vi "ISS Main.vi"() -> ()   [LabVIEW 2014]
uses:
  <vilib>/Instr/_visa.llb/VISA Configure Serial Port (Instr).vi
  controls/scan data action.ctl
  controls/main states.ctl
  <vilib>/Utility/file.llb/Write To Spreadsheet File (DBL).vi
  controls/ADC settings.ctl
  controls/PD settings.ctl
  controls/LD settings.ctl
  controls/temperature sensor.ctl
  controls/general.ctl
panel:
  in  "automatic save":bool
  out "stat time":T1
  in  "Tab Control":enum32{"Scan", "Settings"}(tab)
  out "ADC ratio":dbl[](array[numeric]) format="%#_4g"
  out "XY Graph":T2(graph)
  out "Statistics":T3(array[cluster]) {"mean" format="%#_3g"; "std/mean" format="%#_2e"}
  in  "save":bool
  in  "exit":bool
  in  "stop scan":bool
  in  "start scan":bool
  in  "channels to read":i32[](array[numeric])=[2] min=0 max=3 step=1
  in  "#points to read":i32=36000 min=0 step=1
  out "#points read":i32
  in  "ADC settings":T4={"ADCspeed"=1.0, "ADCgain"=1.0, "ADC Integrate"=1.0, "sampling \nfrequency (Hz)"=1.0}
  in  "Temperature control":T5=["taped next to active fiber to breadboard", "lower left corner of breadboard, away from components", "on temp control", "at former PBS position", "free air above tube"]
  in  "Photodiodes":T6=[{"LD ID"="G12180-120A #2", "Temp. [kOhm]"=47.0, "LD setup"="Tube, no angle, FC/APC"}]
  in  "Laser diode":T7=[{"LD ID"=811007, "Current [mA]"=341.0, "Temperature [V]"=1.1865}, {"LD ID"=811009, "Current [mA]"=308.0, "Temperature [V]"=1.866}]
  in  "PD Current meter":refnum<visa-resource-name>="COM3"
  in  "Temp. monitoring":refnum<visa-resource-name>="COM4"
  in  "read temperature":bool=TRUE
  in  "general information":T8={"Operator"="Philippe", "Setup"="Yb005", "Purpose of measurement"="ca. 2-3mm of Yb198 fiber attached for Yb005, with 1m of CLF, since attached hood to fiber there is some minor pump (100pW)"}
  in  "Path to folder":path=path "V:/labdata and figures/Ytterbium-Setup/ISS-Yb005/Scan3"
  out "current data":dbl[](array[numeric])
  out "appended array":dbl[][](array[numeric])
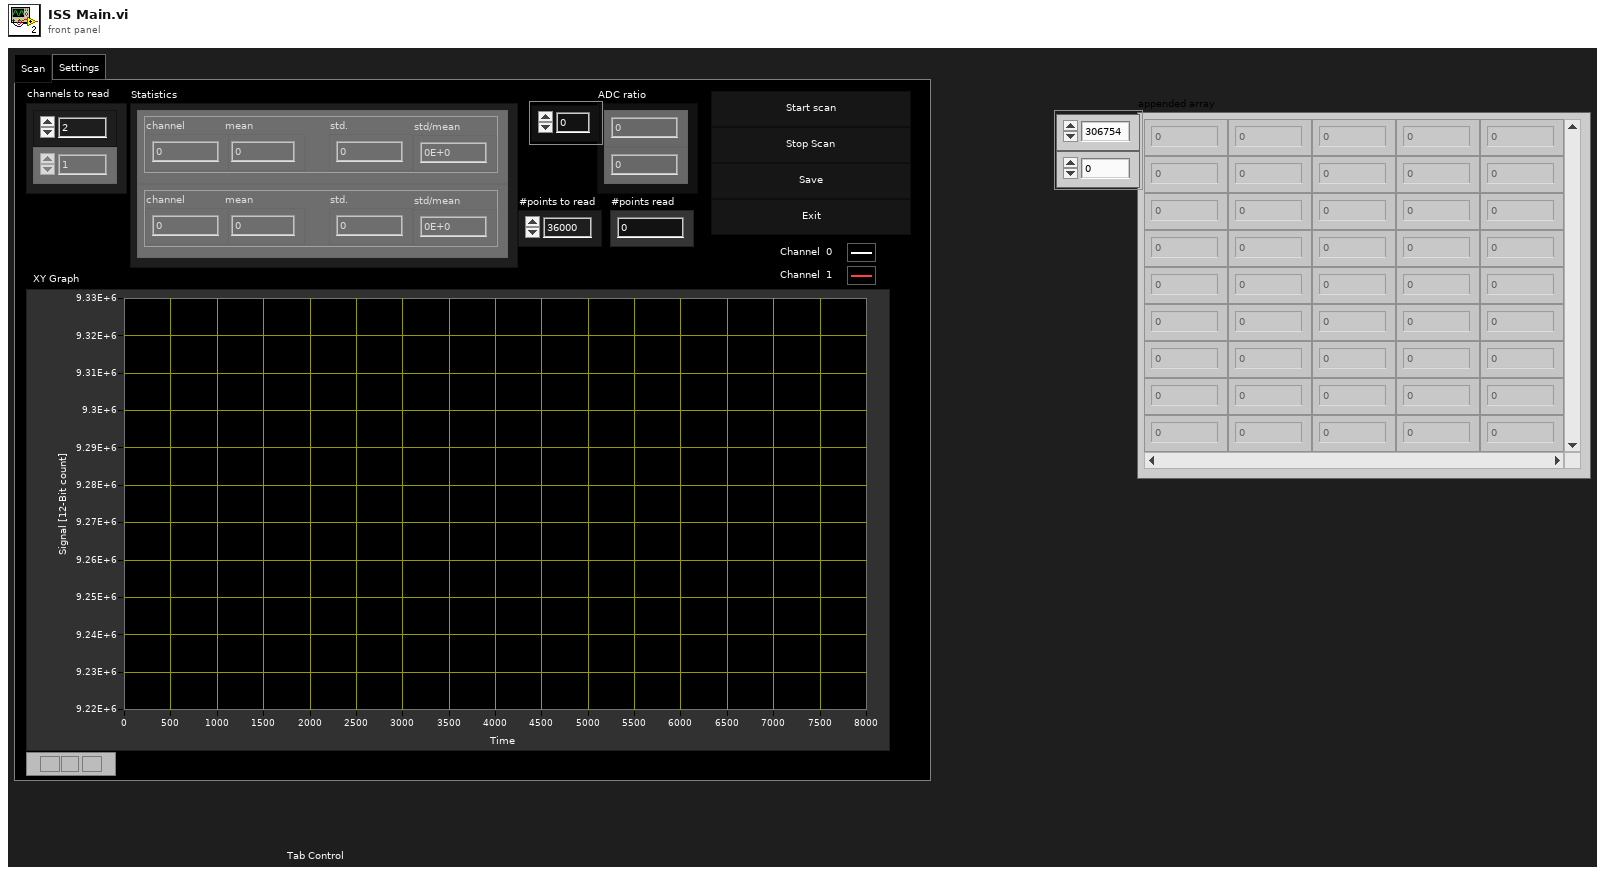
[diagram p1: front panel]
types:
  T1 = cluster{"date string":string, "time string":string}
  T2 = cluster{"Output Data":dbl[], "Output Data":dbl[]}[]
  T3 = cluster{"channel":i32, "mean":dbl, "std.":dbl, "std/mean":dbl}[]
  T4 = typedef "ADC settings.ctl" = cluster{"ADCspeed":dbl, "ADCgain":dbl, "ADC Integrate":dbl, "sampling \nfrequency (Hz)":dbl}
  T5 = typedef "temperature sensor.ctl" = string[]
  T6 = typedef "PD settings.ctl" = cluster{"LD ID":string, "Temp. [kOhm]":dbl, "LD setup":string}[]
  T7 = typedef "LD settings.ctl" = cluster{"LD ID":i32, "Current [mA]":dbl, "Temperature [V]":dbl}[]
  T8 = typedef "general.ctl" = cluster{"Operator":string, "Setup":string, "Purpose of measurement":string}
  T9 = typedef "main states.ctl" = enum16{"Initialize", "Wait for User Input", "exit"}
  T10 = enum8{"Enabled", "Disabled", "Disabled and Grayed Out"}
  T11 = typedef "All Message Queues.ctl" = cluster{"PD Control":refnum<queue>, "temp. reading":refnum<queue>}
  T12 = typedef "main states.ctl" = enum16{"Wait for User Input", "exit"}
  T13 = typedef "scan data action.ctl" = enum16{"initialize", "append", "read", "write"}
  T14 = typedef "Message Queue.lvlib/Message Cluster.ctl" = cluster{"Message":string, "Message Data":variant}
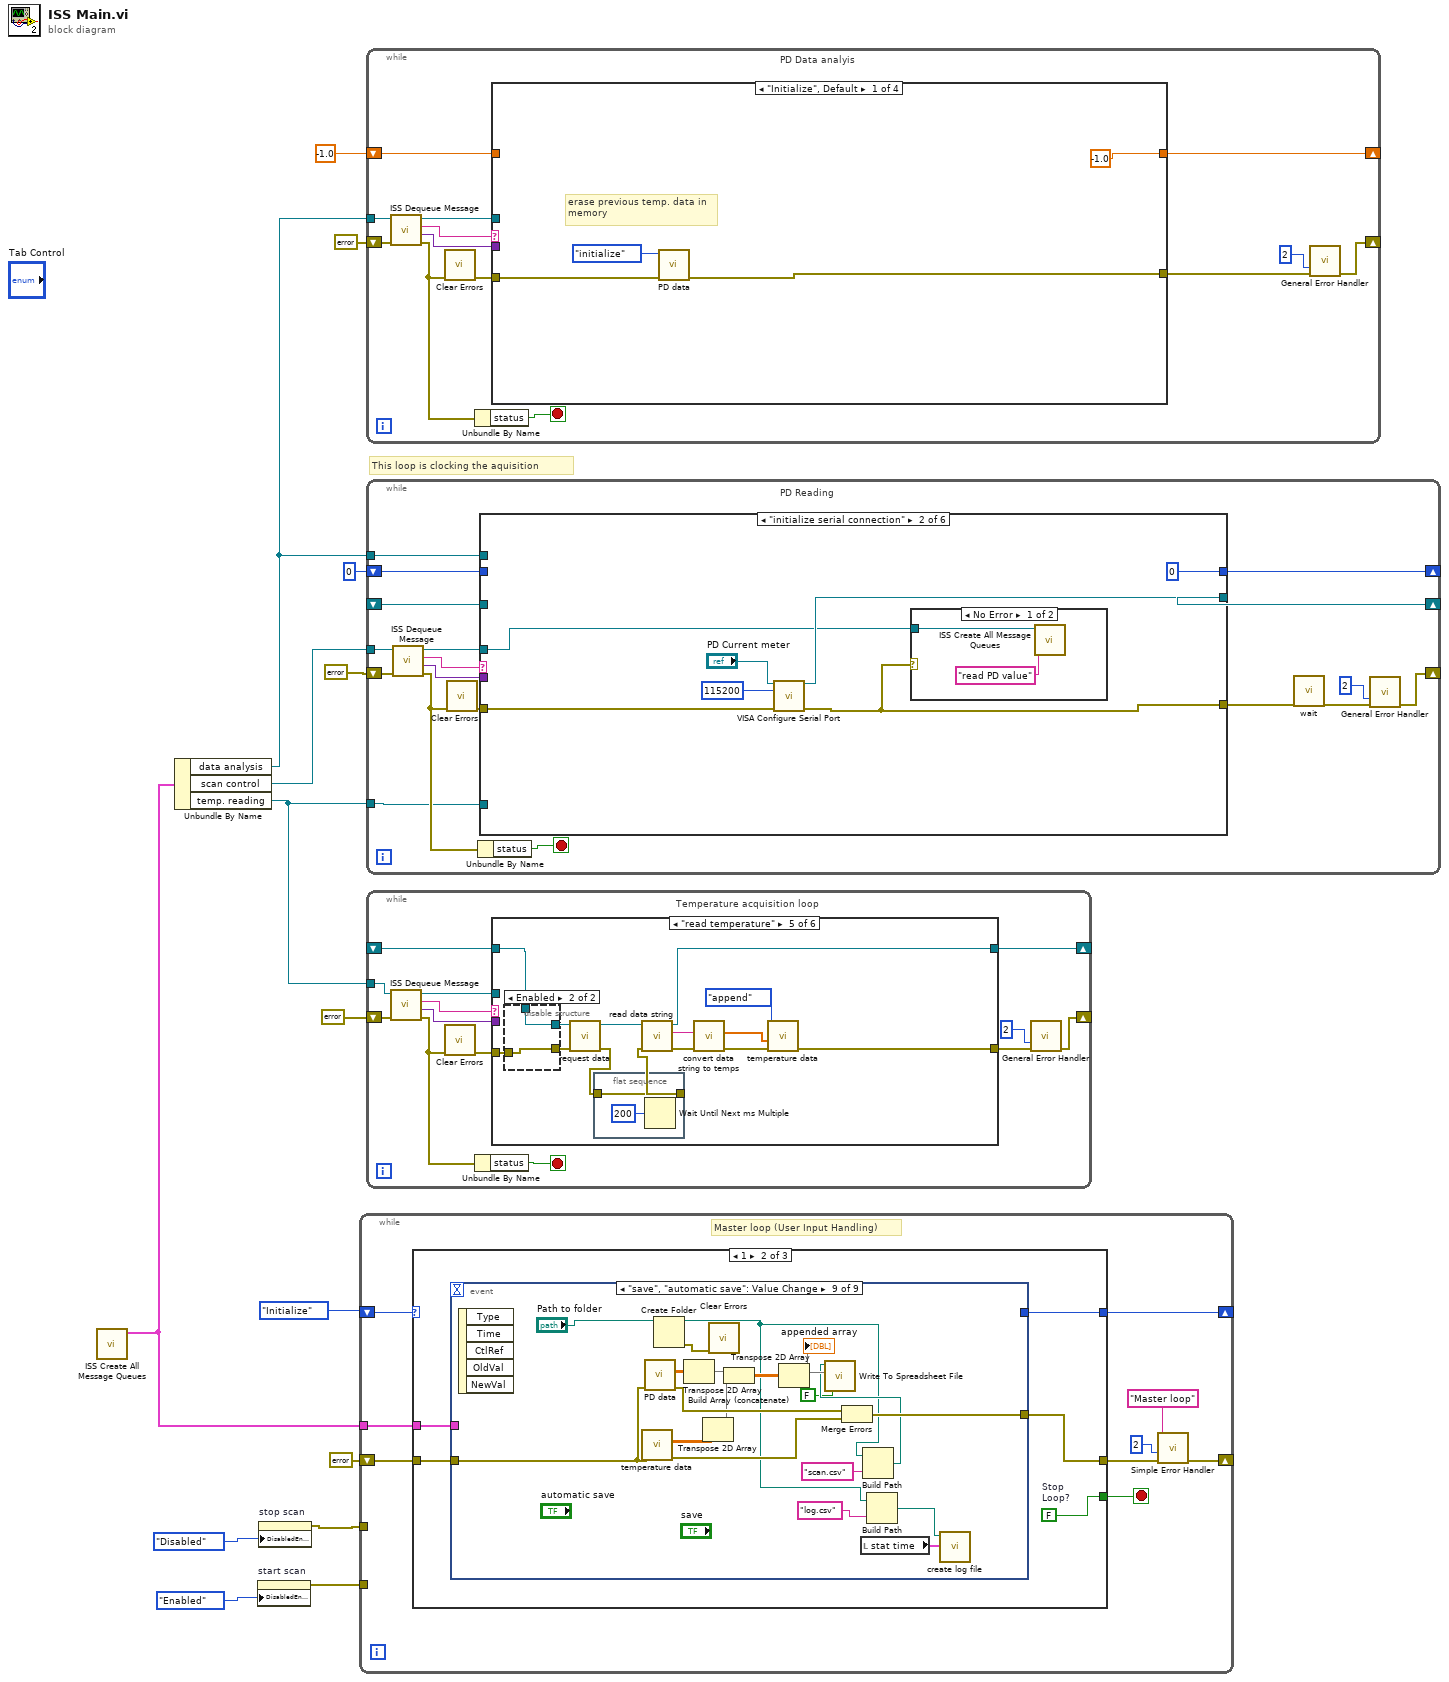
[diagram p0: block diagram]
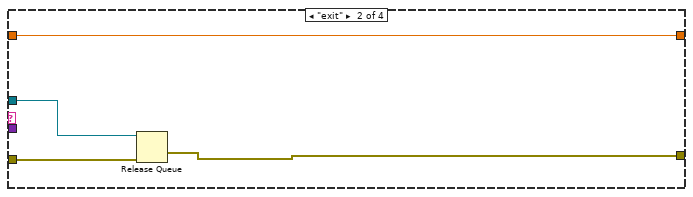
[diagram p2: hidden frame]
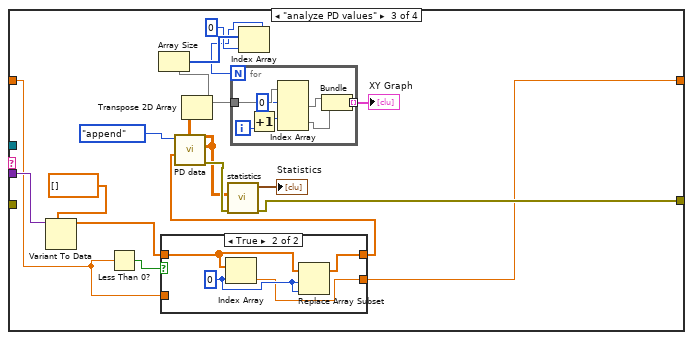
[diagram p3: hidden frame]
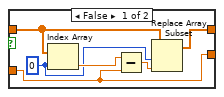
[diagram p4: hidden frame]
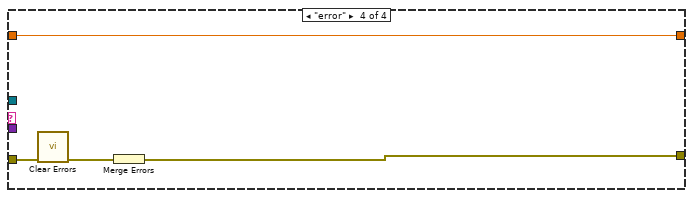
[diagram p5: hidden frame]
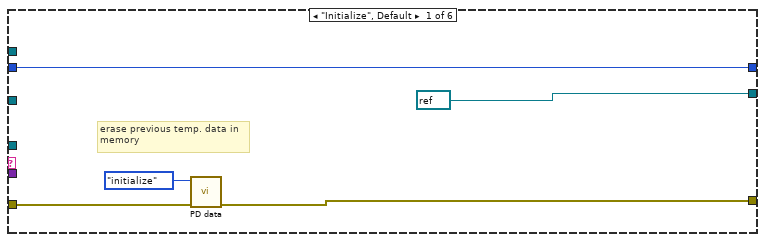
[diagram p6: hidden frame]
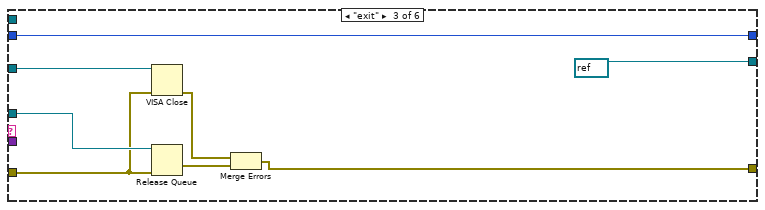
[diagram p8: hidden frame]
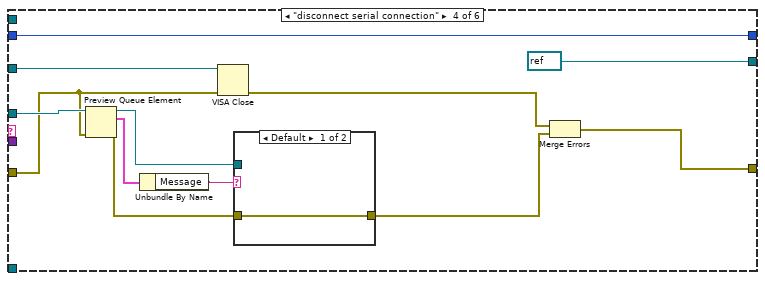
[diagram p9: hidden frame]
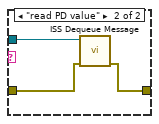
[diagram p10: hidden frame]
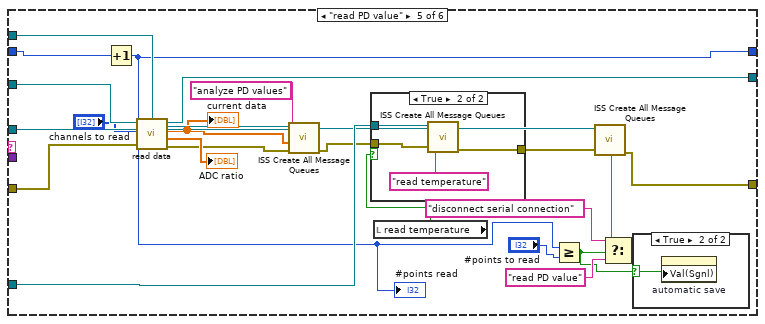
[diagram p11: hidden frame]
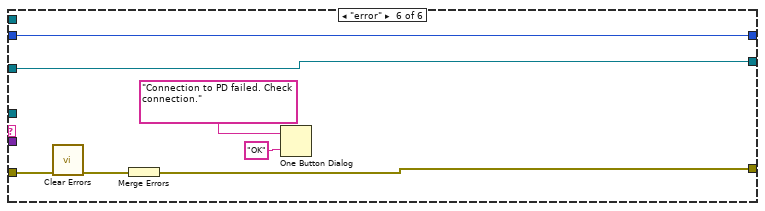
[diagram p14: hidden frame]
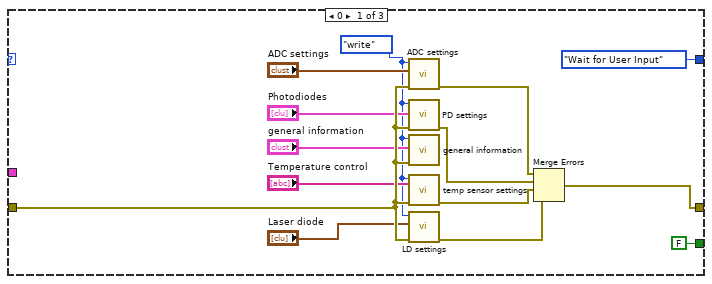
[diagram p15: hidden frame]
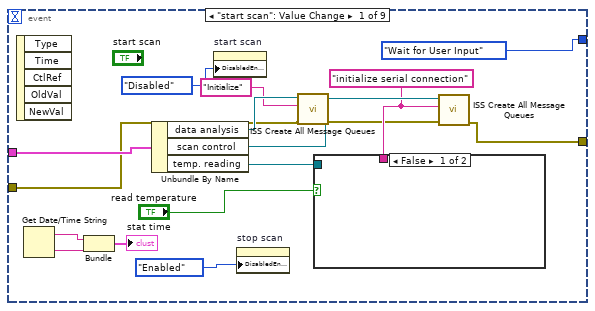
[diagram p16: hidden frame]
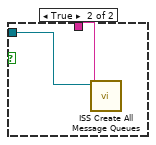
[diagram p17: hidden frame]
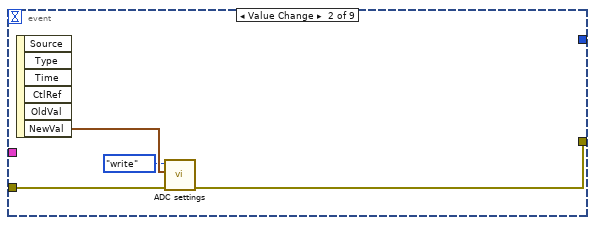
[diagram p18: hidden frame]
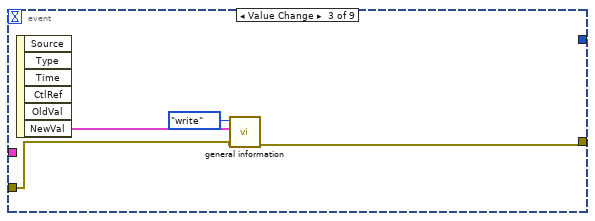
[diagram p19: hidden frame]
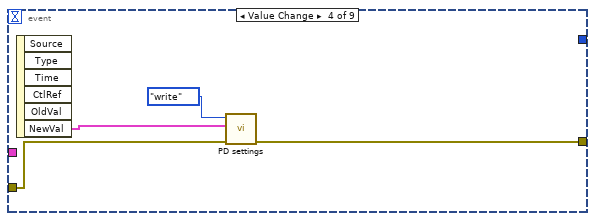
[diagram p20: hidden frame]
diagram:
  # "This loop is clocking the aquisition"
  n1 = call "ISS Create All Message Queues.vi"() -> ("Message Queues out"=w10:T11)  [unwired: 10 in, 1 out]
  n2 = Unbundle By Name(w10) -> ("data analysis"=w2:refnum<queue>, "scan control"=w13:refnum<queue>, "temp. reading"=w12:refnum<queue>)
  n3 = property on="start scan" class="Bool"("DisabledEnum"=T10."Enabled" ("Disabled")) -> (error out=w6:errorcluster)  [unwired: 2 in, 1 out]
  n4 = property on="stop scan" class="Bool"("DisabledEnum"=T10."Disabled" ("Disabled")) -> (error out=w7:errorcluster)  [unwired: 2 in, 1 out]
  n5 = while {
    shift-right: [w23] -> _
    shift-left: main_states."Initialize" ("Initial State") -> [w24]
    shift-right: [w20] -> _
    shift-left: errorcluster {"status"=FALSE, "code"=0, "source"=""} ("error out") -> [w22]
    tunnel: w10 -> [w18]
    tunnel: w7 -> [_]
    tunnel: w6 -> [_]
    stop <- w19 stop-if-true
    # "Master loop (User Input Handling)"
    n6 = case shown="1" w24 {
      tunnel: [main_states."Wait for User Input" ("Initial State") w43 main_states."exit" ("Initial State")] -> w23
      tunnel: [FALSE ("Stop Loop?") w42 w129] -> w19
      tunnel: w22 -> [w38 w41 w124]
      tunnel: [w33 w40 w123] -> w21
      tunnel: w18 -> [_ w39 w127]
      frame 0 {
        w26 = enum16{"read", "write"}."write" ("mode (R)")
        n7 = call "ADC settings.vi"("Error In"=w38, "ADC settings in"="ADC settings", "mode (R)"=w26) -> ("Error out"=w37:errorcluster)  [unwired: 7 in, 1 out]
        n8 = call "PD settings.vi"("Error In"=w38, "PD settings"="Photodiodes", "mode (R)"=w26) -> ("Error out"=w36:errorcluster)  [unwired: 7 in, 1 out]
        n9 = call "general information.vi"("Error In"=w38, "General information in"="general information", "mode (R)"=w26) -> ()  [unwired: 7 in, 2 out]
        n10 = call "temp sensor settings.vi"("Error In"=w38, "temperature sensor information"="Temperature control", "mode (R)"=w26) -> ("Error out"=w35:errorcluster)  [unwired: 7 in, 1 out]
        n11 = call "LD settings.vi"("Error In"=w38, "General information in"="Laser diode", "mode (R)"=w26) -> ("Error out"=w34:errorcluster)  [unwired: 7 in, 1 out]
        n12 = Merge Errors(w37, w36, w35, w34) -> (w33:errorcluster)
      }
      frame 1 {
        w42 = FALSE  # Stop  Loop?
        n13 = event shown="[8] \"save\", \"automatic save\": Value Change" {
          selector: _ -> [_ _ _ _ _ _ _ _ _]
          dyn-events: _ -> [_ _ _ _ _ _ _ _ _]
          timeout: _ -> [_ _ _ _ _ _ _ _ _]
          tunnel: [main_states."Wait for User Input" ("Initial State") _ _ _ _ _ main_states."Wait for User Input" ("Initial State") main_states."exit" ("Initial State") _] -> w43
          tunnel: w41 -> [w49 w63 w69 w71 w76 w80 w87 w94 w120]
          tunnel: [w53 w62 w68 w70 w75 w79 w84 w93 w117] -> w40
          tunnel: w39 -> [w58 _ _ _ _ _ w91 w96 _]
          event "start scan": Value Change {
            w54 = "initialize serial connection" ("Message")
            n14 = event-data() -> ()  [unwired: 1 in, 5 out]
            n15 = Get Date/Time String() -> (date string=w45:string, time string=w46:string)  [unwired: 3 in]
            n16 = Bundle("date string"=w45, "time string"=w46) -> (→"stat time":T1)  [unwired: 1 in]
            n17 = Unbundle By Name(w58) -> ("data analysis"=w50:refnum<queue>, "scan control"=w57:refnum<queue>, "temp. reading"=w56:refnum<queue>)
            n18 = property on="start scan" class="Bool"("DisabledEnum"=T10."Disabled" ("Disabled")) -> ()  [unwired: 2 in, 2 out]
            n19 = property on="stop scan" class="Bool"("DisabledEnum"=T10."Enabled" ("Disabled")) -> ()  [unwired: 2 in, 2 out]
            n20 = call "ISS Create All Message Queues.vi"("error in (no error)"=w49, 10:"Initialize" ("Message"), 11:w50) -> ("error out"=w48:errorcluster)  [unwired: 7 in, 1 out]
            n21 = case shown="False" "read temperature" {
              tunnel: w56 -> [_ w61]
              tunnel: w54 -> [_ w60]
              frame False {
              }
              frame True {
                n22 = call "ISS Create All Message Queues.vi"(10:w60, 11:w61) -> ()  [unwired: 8 in, 2 out]
              }
            }
            n23 = call "ISS Create All Message Queues.vi"("error in (no error)"=w48, 10:w54, 11:w57) -> ("error out"=w53:errorcluster)  [unwired: 7 in, 1 out]
          }
          event Value Change {
            n24 = event-data() -> ("NewVal"=w65:T4)  [unwired: 1 in, 5 out]
            n25 = call "ADC settings.vi"("Error In"=w63, "ADC settings in"=w65, "mode (R)"=enum16{"read", "write"}."write") -> ("Error out"=w62:errorcluster)  [unwired: 7 in, 1 out]
          }
          event Value Change {
            n26 = event-data() -> ("NewVal"=w67:T8)  [unwired: 1 in, 5 out]
            n27 = call "general information.vi"("Error In"=w69, "General information in"=w67, "mode (R)"=enum16{"read", "write"}."write") -> ("Error out"=w68:errorcluster)  [unwired: 7 in, 1 out]
          }
          event Value Change {
            n28 = event-data() -> ("NewVal"=w73:T6)  [unwired: 1 in, 5 out]
            n29 = call "PD settings.vi"("Error In"=w71, "PD settings"=w73, "mode (R)"=enum16{"read", "write"}."write") -> ("Error out"=w70:errorcluster)  [unwired: 7 in, 1 out]
          }
          event Value Change {
            n30 = event-data() -> ("NewVal"=w77:T7)  [unwired: 1 in, 5 out]
            n31 = call "LD settings.vi"("Error In"=w76, "General information in"=w77, "mode (R)"=enum16{"read", "write"}."write") -> ("Error out"=w75:errorcluster)  [unwired: 7 in, 1 out]
          }
          event Value Change {
            n32 = event-data() -> ("NewVal"=w78:T5)  [unwired: 1 in, 5 out]
            n33 = call "temp sensor settings.vi"("Error In"=w80, "temperature sensor information"=w78) -> ("Error out"=w79:errorcluster)  [unwired: 8 in, 1 out]
          }
          event "stop scan": Value Change {
            w88 = "disconnect serial connection" ("Message")
            n34 = event-data() -> ()  [unwired: 1 in, 5 out]
            n35 = Unbundle By Name(w91) -> ("scan control"=w90:refnum<queue>, "temp. reading"=w89:refnum<queue>)
            n36 = call "ISS Create All Message Queues.vi"("error in (no error)"=w87, 10:w88, 11:w90) -> ("error out"=w85:errorcluster)  [unwired: 7 in, 1 out]
            n37 = call "ISS Create All Message Queues.vi"("error in (no error)"=w87, 10:w88, 11:w89) -> ("error out"=w86:errorcluster)  [unwired: 7 in, 1 out]
            n38 = Merge Errors(w85, w86) -> (w84:errorcluster)
            n39 = property on="stop scan" class="Bool"("DisabledEnum"=T10."Disabled" ("Disabled")) -> ()  [unwired: 2 in, 2 out]
            n40 = property on="start scan" class="Bool"("DisabledEnum"=T10."Enabled" ("Disabled")) -> ()  [unwired: 2 in, 2 out]
          }
          event "exit": Value Change {
            n41 = event-data() -> ()  [unwired: 1 in, 5 out]
            n42 = Cluster To Array(cluster=w96) -> (array=w95:refnum<queue>[])
            n43 = for {
              tunnel: w95 -> [w103] mode=indexing
              shift-right: [w97] -> w93
              shift-left: w94 -> [w99]
              n44 = call "ISS Create All Message Queues.vi"("error in (no error)"=w99, 10:"disconnect serial connection" ("Message"), 11:w103) -> ("error out"=w100:errorcluster, "Message Queues out"=w101:T11)  [unwired: 7 in]
              n45 = call "ISS Create All Message Queues.vi"("error in (no error)"=w100, 10:"exit" ("Message"), 11:w101) -> ("error out"=w97:errorcluster)  [unwired: 7 in, 1 out]
            }
          }
          event "save", "automatic save": Value Change {
            n46 = event-data() -> ()  [unwired: 1 in, 5 out]
            n47 = call "temperature data.vi"("Error In"=w120) -> ("Error out"=w118:errorcluster, "Output Data"=w121:dbl[][])  [unwired: 9 in]
            n48 = call "PD data.vi"("Error In"=w120) -> ("Error out"=w119:errorcluster, "Output Data"=w122:dbl[][])  [unwired: 9 in]
            n49 = Create Folder(path (use dialog)="Path to folder") -> (created path=w106:path, error out=w105:errorcluster)  [unwired: 2 in, 1 out]
            n50 = Transpose 2D Array(2D array=w122) -> (transposed array=w115:dbl[][])
            n51 = Transpose 2D Array(2D array=w121) -> (transposed array=w113:dbl[][])
            n52 = call <vilib>:"Clear Errors.vi"("error in (no error)"=w105) -> ()  [unwired: 5 in, 2 out]
            n53 = Build Array (concatenate)(w115, w113) -> (w116:dbl[][])
            n54 = Transpose 2D Array(2D array=w116) -> (transposed array=w114:dbl[][])
            "appended array" <- w114
            n55 = Merge Errors(w119, w118) -> (w117:errorcluster)
            n56 = local read "stat time"() -> (w112:T1)
            n57 = Build Path(base path=w106, name or relative path="scan.csv") -> (appended path=w110:path)
            n58 = call-poly <vilib>:"Write To Spreadsheet File.vi"("append to file? (new file:F)"=FALSE, "2D data"=w114, "file path (dialog if empty)"=w110) -> ()  [unwired: 5 in, 1 out]
            n59 = Build Path(base path=w106, name or relative path="log.csv") -> (appended path=w108:path)
            n60 = call "create log file.vi"("stat time"=w112, "config file path"=w108) -> ()  [unwired: 9 in, 1 out]
          }
        }
      }
      frame 2 {
        w129 = TRUE  # Stop Loop?
        # "Exit - Exit the application."
        n61 = Cluster To Array(cluster=w127) -> (array=w126:refnum<queue>[])
        n62 = for {
          tunnel: w126 -> [w132] mode=indexing
          tunnel: "exit" ("Message") -> [w133]
          shift-right: [w131] -> w123
          shift-left: w124 -> [w130]
          n63 = call "ISS Create All Message Queues.vi"("error in (no error)"=w130, 10:w133, 11:w132) -> ("error out"=w131:errorcluster)  [unwired: 7 in, 1 out]
        }
      }
    }
    n64 = call <vilib>:"Simple Error Handler.vi"("error source (\" \")"="Master loop" ("error source (\" \")"), "type of dialog (OK msg:1)"=2, "error in (no error)"=w21) -> ("error out"=w20:errorcluster)  [unwired: 2 in, 4 out]
  }
  n65 = while "PD Data analyis" {
    shift-right: [w142] -> _
    shift-left: errorcluster {"status"=FALSE, "code"=0, "source"=""} ("error out") -> [w144]
    tunnel: w2 -> [w137]
    shift-right: [w134] -> _
    shift-left: -1.0 ("Numeric Control") -> [w135]
    stop <- w139 stop-if-true
    n66 = call "ISS Dequeue Message.vi"("error in (no error)"=w144, "Message Queue"=w137) -> ("error out"=w145:errorcluster, "Message Data"=w140:variant, "Message"=w146:string, "dup Message Queue"=w143:refnum<queue>)  [unwired: 6 in]
    n67 = call <vilib>:"Clear Errors.vi"("error in (no error)"=w145) -> ("error out"=w138:errorcluster)  [unwired: 5 in, 1 out]
    n68 = Unbundle By Name(w145) -> ("status"=w139:bool)
    n69 = case shown="\"Initialize\", Default" w146 {
      tunnel: w138 -> [w150 w153 _ w192]
      tunnel: [w149 w152 w160 w191] -> w136
      tunnel: w143 -> [_ w154 _ _]
      tunnel: w140 -> [_ _ w164 _]
      tunnel: w135 -> [_ w151 w156 w189]
      tunnel: [-1.0 ("Numeric Control") w151 w158 w189] -> w134
      frame "Initialize", Default {
        # "erase previous temp. data in\nmemory"
        n70 = call "PD data.vi"("Error In"=w150, "mode (R)"=scan_data_action."initialize") -> ("Error out"=w149:errorcluster)  [unwired: 8 in, 1 out]
      }
      frame "exit" {
        n71 = Release Queue(queue=w154, error in (no error)=w153) -> (error out=w152:errorcluster)  [unwired: 1 in, 2 out]
      }
      frame "analyze PD values" {
        n72 = Variant To Data(type=dbl[] [] ("data"), Variant=w164) -> (data=w159:dbl[])  [unwired: 1 in, 1 out]
        n73 = Less Than 0?(x=w156) -> (x < 0?=w155:bool)
        n74 = case shown="True" w155 {
          tunnel: w159 -> [w174 w180]
          tunnel: [w172 w178] -> w158
          tunnel: [w173 w179] -> w157
          tunnel: w156 -> [w172 _]
          frame False {
            w175 = 0 ("index")
            n75 = Index Array(array=w174, index=w175) -> (element=w177:dbl)
            n76 = Subtract(x=w177, y=w172) -> (x-y=w176:dbl)
            n77 = Replace Array Subset(array=w174, new element=w176, index=w175) -> (w173:dbl[])
          }
          frame True {
            w181 = 0 ("index")
            n78 = Index Array(array=w180, index=w181) -> (element=w178:dbl)
            n79 = Replace Array Subset(array=w180, new element=w181, index=w181) -> (w179:dbl[])
          }
        }
        n80 = call "PD data.vi"("append element"=w157, "mode (R)"=scan_data_action."append") -> ("Error out"=w170:errorcluster, "Output Data"=w166:dbl[][])  [unwired: 8 in]
        n81 = Transpose 2D Array(2D array=w166) -> (transposed array=w167:dbl[][])
        n82 = Array Size(array=w167) -> (size(s)=w169:i32[])
        n83 = call "statistics.vi"("Error In"=w170, "Data"=w166) -> ("Error Out"=w160:errorcluster, "Statistics"=→"Statistics":T3)  [unwired: 8 in]
        n84 = Index Array(array=w169, index=0) -> (element=w165:i32)
        n85 = for {
          N: w165 -> [_]
          tunnel: w167 -> [w188]
          tunnel: [w182] -> w162 mode=indexing
          i -> [w186]
          n86 = Increment(x=w186) -> (x+1=w185:i32)
          n87 = Index Array(array=w188, index (row) #1=0 ("index (row)"), index (row) #2=w185) -> (element #1=w184:dbl[], element #2=w183:dbl[])  [unwired: 2 in]
          n88 = Bundle(w184, w183) -> (w182:cluster{dbl[], dbl[]})  [unwired: 1 in]
        }
        "XY Graph" <- w162
      }
      frame "error" {
        n89 = call <vilib>:"Clear Errors.vi"("error in (no error)"=w192) -> ("error out"=w190:errorcluster)  [unwired: 5 in, 1 out]
        n90 = Merge Errors(w190) -> (w191:errorcluster)
      }
    }
    n91 = call <vilib>:"General Error Handler.vi"("type of dialog (OK msg:1)"=2, "error in (no error)"=w136) -> ("error out"=w142:errorcluster)  [unwired: 9 in, 4 out]
  }
  n92 = while "PD Reading" {
    shift-right: [w206] -> _
    shift-left: errorcluster {"status"=FALSE, "code"=0, "source"=""} ("error constant") -> [w208]
    shift-right: [w201] -> _
    shift-left: _ -> [w200]
    tunnel: w13 -> [w199]
    tunnel: w12 -> [w198]
    shift-right: [w193] -> _
    shift-left: 0 ("channel to read") -> [w195]
    tunnel: w2 -> [w194]
    stop <- w203 stop-if-true
    n93 = call "ISS Dequeue Message.vi"("error in (no error)"=w208, "Message Queue"=w199) -> ("error out"=w209:errorcluster, "Message Data"=w204:variant, "Message"=w210:string, "dup Message Queue"=w207:refnum<queue>)  [unwired: 6 in]
    n94 = call <vilib>:"Clear Errors.vi"("error in (no error)"=w209) -> ("error out"=w202:errorcluster)  [unwired: 5 in, 1 out]
    n95 = Unbundle By Name(w209) -> ("status"=w203:bool)
    n96 = case shown="\"initialize serial connection\"" w210 {
      tunnel: w202 -> [w215 w218 w229 w235 w269 w281]
      tunnel: [w214 w216 w226 w236 w265 w280] -> w197
      tunnel: w207 -> [_ w219 w232 w243 w266 _]
      tunnel: w204 -> [_ _ _ _ _ _]
      tunnel: [refnum<visa-resource-name> refnum ("VISA Resource out") w221 refnum<visa-resource-name> refnum ("VISA Refnum out") refnum<visa-resource-name> refnum ("VISA resource name out") w268 w279] -> w201
      tunnel: w200 -> [_ _ w231 w234 w270 w279]
      tunnel: w198 -> [_ _ _ _ w267 _]
      tunnel: w195 -> [w211 _ w225 w233 w257 w277]
      tunnel: w194 -> [_ _ _ _ w253 _]
      tunnel: [w211 0 ("channel to read") w225 w233 w250 w277] -> w193
      frame "Initialize", Default {
        # "erase previous temp. data in\nmemory"
        n97 = call "PD data.vi"("Error In"=w215, "mode (R)"=scan_data_action."initialize") -> ("Error out"=w214:errorcluster)  [unwired: 8 in, 1 out]
      }
      frame "initialize serial connection" {
        n98 = call-poly "VISA Configure Serial Port"("VISA resource name"="PD Current meter", "baud rate (9600)"=u32 115200, "error in (no error)"=w218) -> ("VISA resource name out"=w221:refnum<visa-resource-name>, "error out"=w216:errorcluster)  [unwired: 11 in]
        n99 = case shown="No Error" w216 {
          tunnel: w219 -> [w223 _]
          frame No Error {
            n100 = call "ISS Create All Message Queues.vi"(10:"read PD value" ("notification"), 11:w223) -> ()  [unwired: 8 in, 2 out]
          }
          frame Error {
          }
        }
      }
      frame "exit" {
        n101 = VISA Close(VISA resource name=w231, error in (no error)=w229) -> (error out=w228:errorcluster)
        n102 = Release Queue(queue=w232, error in (no error)=w229) -> (error out=w227:errorcluster)  [unwired: 1 in, 2 out]
        n103 = Merge Errors(w228, w227) -> (w226:errorcluster)
      }
      frame "disconnect serial connection" {
        n104 = Preview Queue Element(queue=w243, error in (no error)=w235) -> (queue out=w240:refnum<queue>, element=w242:T14, error out=w239:errorcluster)  [unwired: 1 in, 1 out]
        n105 = Unbundle By Name(w242) -> ("Message"=w241:string)
        n106 = VISA Close(VISA resource name=w234, error in (no error)=w235) -> (error out=w237:errorcluster)
        n107 = case shown="Default" w241 {
          tunnel: w240 -> [_ w248]
          tunnel: w239 -> [w245 w247]
          tunnel: [w245 w246] -> w238
          frame Default {
          }
          frame "read PD value" {
            n108 = call "ISS Dequeue Message.vi"("error in (no error)"=w247, "Message Queue"=w248) -> ("error out"=w246:errorcluster)  [unwired: 6 in, 3 out]
          }
        }
        n109 = Merge Errors(w237, w238) -> (w236:errorcluster)
      }
      frame "read PD value" {
        n110 = Increment(x=w257) -> (x+1=w250:i32)
        "#points read" <- w250
        n111 = call "read data.vi"("error in (no error)"=w269, "channels to read"="channels to read", "VISA Refnum in"=w270) -> ("error out"=w255:errorcluster, "ADC ratio"=→"ADC ratio":dbl[], "data"=w252:dbl[], "VISA Refnum out"=w268:refnum<visa-resource-name>)  [unwired: 4 in, 1 out]
        "current data" <- w252
        n112 = call "ISS Create All Message Queues.vi"("error in (no error)"=w255, 9:w252, 10:"analyze PD values" ("Message"), 11:w253) -> ("error out"=w254:errorcluster)  [unwired: 6 in, 1 out]
        n113 = local read "read temperature"() -> (w264:bool)
        n114 = case shown="True" w264 {
          tunnel: w267 -> [_ w276]
          tunnel: w254 -> [w272 w274]
          tunnel: [w272 w273] -> w256
          frame False {
          }
          frame True {
            n115 = call "ISS Create All Message Queues.vi"("error in (no error)"=w274, 10:"read temperature" ("notification"), 11:w276) -> ("error out"=w273:errorcluster)  [unwired: 7 in, 1 out]
          }
        }
        n116 = Greater Or Equal?(x=w250, y="#points to read") -> (x >= y?=w249:bool)
        n117 = Select(t="disconnect serial connection" ("notification"), s=w249, f="read PD value" ("notification")) -> (s? t:f=w259:string)
        n118 = call "ISS Create All Message Queues.vi"("error in (no error)"=w256, 10:w259, 11:w266) -> ("error out"=w265:errorcluster)  [unwired: 7 in, 1 out]
        n119 = case shown="True" w249 {
          selector: w249 -> [_ w271]
          frame False {
          }
          frame True {
            n120 = property on="automatic save" class="Bool (strict)"("Val(Sgnl)"=w271) -> ()  [unwired: 2 in, 2 out]
          }
        }
      }
      frame "error" {
        n121 = call <vilib>:"Clear Errors.vi"("error in (no error)"=w281) -> ("error out"=w278:errorcluster)  [unwired: 5 in, 1 out]
        n122 = Merge Errors(w278) -> (w280:errorcluster)
        n123 = One Button Dialog(message="Connection to PD failed. Check connection.", button name ("OK")="OK") -> ()  [unwired: 1 out]
      }
    }
    n124 = call "wait.vi"("Error In"=w197) -> ("Error Out"=w196:errorcluster)  [unwired: 10 in]
    n125 = call <vilib>:"General Error Handler.vi"("type of dialog (OK msg:1)"=2, "error in (no error)"=w196) -> ("error out"=w206:errorcluster)  [unwired: 9 in, 4 out]
  }
  n126 = while "Temperature acquisition loop" {
    shift-right: [w291] -> _
    shift-left: errorcluster {"status"=FALSE, "code"=0, "source"=""} ("error constant") -> [w294]
    shift-right: [w286] -> _
    shift-left: _ -> [w285]
    tunnel: w12 -> [w284]
    stop <- w288 stop-if-true
    n127 = call "ISS Dequeue Message.vi"("error in (no error)"=w294, "Message Queue"=w284) -> ("error out"=w295:errorcluster, "Message Data"=w289:variant, "Message"=w296:string, "dup Message Queue"=w293:refnum<queue>)  [unwired: 6 in]
    n128 = call <vilib>:"Clear Errors.vi"("error in (no error)"=w295) -> ("error out"=w287:errorcluster)  [unwired: 5 in, 1 out]
    n129 = Unbundle By Name(w295) -> ("status"=w288:bool)
    n130 = case shown="\"read temperature\"" w296 {
      tunnel: w287 -> [w300 w306 w310 w319 w333 w353]
      tunnel: [w299 w308 w309 w313 w335 w352] -> w292
      tunnel: w293 -> [_ _ w312 w318 _ _]
      tunnel: w289 -> [_ _ _ _ _ _]
      tunnel: [refnum<visa-resource-name> refnum ("VISA Resource out") w307 w311 refnum<visa-resource-name> refnum ("VISA resource name out") w338 w351] -> w286
      tunnel: w285 -> [_ _ w311 w323 w332 w351]
      frame "Initialize", Default {
        # "erase previous temp. data in\nmemory"
        n131 = call "temperature data.vi"("Error In"=w300, "mode (R)"=scan_data_action."initialize") -> ("Error out"=w299:errorcluster)  [unwired: 8 in, 1 out]
      }
      frame "initialize serial connection" {
        n132 = call "temperature data.vi"("Error In"=w306, "mode (R)"=scan_data_action."initialize") -> ("Error out"=w304:errorcluster)  [unwired: 8 in, 1 out]
        n133 = call-poly "VISA Configure Serial Port"("VISA resource name"="Temp. monitoring", "Enable Termination\nChar (T)"=FALSE ("Enable Termination\nChar (T)"), "baud rate (9600)"=u32 115200, "error in (no error)"=w304) -> ("VISA resource name out"=w307:refnum<visa-resource-name>, "error out"=w308:errorcluster)  [unwired: 10 in]
      }
      frame "exit" {
        (unwired) TRUE ("status")
        n134 = Release Queue(queue=w312, error in (no error)=w310) -> (error out=w309:errorcluster)  [unwired: 1 in, 2 out]
      }
      frame "disconnect serial connection" {
        n135 = Preview Queue Element(queue=w318, error in (no error)=w319) -> (queue out=w316:refnum<queue>, element=w317:T14, error out=w320:errorcluster)  [unwired: 1 in, 1 out]
        n136 = Unbundle By Name(w317) -> ("Message"=w321:string)
        n137 = VISA Close(VISA resource name=w323, error in (no error)=w319) -> (error out=w315:errorcluster)
        n138 = case shown="\"read temperature\"" w321 {
          tunnel: w316 -> [_ w327]
          tunnel: w320 -> [w324 w326]
          tunnel: [w324 w325] -> w314
          frame Default {
          }
          frame "read temperature" {
            n139 = call "ISS Dequeue Message.vi"("error in (no error)"=w326, "Message Queue"=w327) -> ("error out"=w325:errorcluster)  [unwired: 6 in, 3 out]
          }
        }
        n140 = Merge Errors(w315, w314) -> (w313:errorcluster)
      }
      frame "read temperature" {
        n141 = disable-structure shown="Enabled" {
          disable-tunnel: w333 -> [w345 w346]
          disable-tunnel: w332 -> [w344 w347]
          disable-tunnel: [w343 w347] -> w331
          disable-tunnel: [w342 w346] -> w330
          frame Disabled {
            n142 = VISA Clear(VISA resource name=w344, error in (no error)=w345) -> (VISA resource name out=w343:refnum<visa-resource-name>, error out=w342:errorcluster)
          }
          frame Enabled {
          }
        }
        n143 = call "request data.vi"("error in"=w330, "VISA resource in"=w331) -> ("error out"=w329:errorcluster, "VISA resource out"=w341:refnum<visa-resource-name>)  [unwired: 8 in]
        n144 = flat-sequence {
          tunnel: w329 -> [w349]
          tunnel: [w349] -> w328
          frame #0 {
            n145 = Wait Until Next ms Multiple(millisecond multiple=u32 200) -> ()  [unwired: 1 out]
          }
        }
        n146 = call "read data string.vi"("error in"=w328, "VISA resource in"=w341) -> ("error out"=w339:errorcluster, "Data string"=w340:string, "VISA Resource out"=w338:refnum<visa-resource-name>)  [unwired: 7 in]
        n147 = call "convert data string to temps.vi"("error in"=w339, "string"=w340) -> ("error out"=w337:errorcluster, "Temperatures"=w334:dbl[])  [unwired: 8 in]
        n148 = call "temperature data.vi"("Error In"=w337, "append element"=w334, "mode (R)"=scan_data_action."append") -> ("Error out"=w335:errorcluster)  [unwired: 7 in, 1 out]
      }
      frame "error" {
        n149 = call <vilib>:"Clear Errors.vi"("error in (no error)"=w353) -> ("error out"=w350:errorcluster)  [unwired: 5 in, 1 out]
        n150 = Merge Errors(w350) -> (w352:errorcluster)
        n151 = One Button Dialog(message="Connection to temp. logger failed. Check connection.", button name ("OK")="OK") -> ()  [unwired: 1 out]
      }
    }
    n152 = call <vilib>:"General Error Handler.vi"("type of dialog (OK msg:1)"=2, "error in (no error)"=w292) -> ("error out"=w291:errorcluster)  [unwired: 9 in, 4 out]
  }
